vi "Obtain servicio from paquetes.vi"(8 "error in (no error)":errorcluster, 10 "Servicio seleccionado":string, 11 "UI in":refnum<class "UI.lvclass">) -> (0 "error out":errorcluster, 3 "UI out":refnum<class "UI.lvclass">)   [LabVIEW 2020, in "UI.lvlib" / "UI.lvclass"]
uses:
  UI.lvclass
  UI.lvclass/UI.ctl
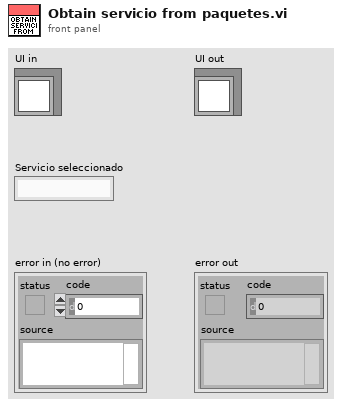
[diagram p1: front panel]
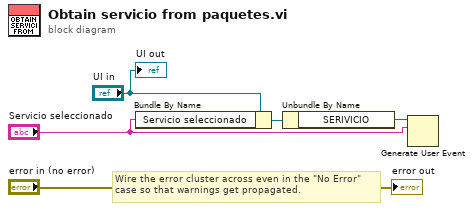
[diagram p0: block diagram]
diagram:
  # "Wire the error cluster across even in the \"No Error\"\ncase so that warnings get propagated."
  n1 = Bundle By Name(cluster="UI in", "Servicio seleccionado"="Servicio seleccionado") -> (w4:refnum<class "UI.lvclass">)
  n2 = Unbundle By Name(w4) -> ("SERIVICIO"=w3:refnum<user-event>)
  n3 = Generate User Event(user event=w3, event data cluster="Servicio seleccionado") -> ()  [unwired: 2 in, 2 out]
  "error out" <- "error in (no error)"
  "UI out" <- "UI in"
